vi "Test String To Codepoint Array.vi"(8 "error in (no error)":errorcluster) -> (0 "error out":errorcluster, 3 "Pass?":bool)   [LabVIEW 2020]
uses:
  G-Unicode/Unicode/Controls/String Encoding.ctl
  G-Unicode/Types/UTF-8 String/UTF-8 String.lvclass/UTF-8 String.ctl
  d266910f-e59a-4c09-865c-c189f5680185.vi
  58239b0c-a6dd-4acd-8f33-f6b76af51e62.vi
  18196cac-081f-454a-8ece-801215b674c5.vi
  G-Unicode/Unicode/Encode String.vi
  d266910f-e59a-4c09-865c-c189f5680185.vi/46bf550a-28c6-4dfd-813a-9b0ad34779ef.vi
  G-Unicode/Private/Conversion/String as Encoded String.vi
  G-Unicode/Private/Conversion/Polymorphic VIs/String as Encoded String (UTF-8 String).vi
  G-Unicode/Types/UTF-8 String/Write Encoded UTF-8 String.vi
  G-Unicode/Private/Library/gu_string_to_codepoint_array.vi
  G-Unicode/Private/Library/gu_codepoint_array_to_string.vi
  G-Unicode/Private/Conversion/Polymorphic VIs/String as Encoded String (LabVIEW String).vi
  G-Unicode/Private/Conversion/Text to UTF-8.vi
  G-Unicode/Private/Conversion/Polymorphic VIs/Text to UTF-8 (LabVIEW String).vi
  G-Unicode/Private/Conversion/Encoded UTF-8 String to Encoded UTF-16LE String.vi
  G-Unicode/Unicode/SubVIs/UTF-16 Byte Swap.vi
  G-Unicode/Private/Conversion/UTF-8 to Text.vi
  G-Unicode/Private/Conversion/Polymorphic VIs/UTF-8 to Text (LabVIEW String).vi
  G-Unicode/Private/Conversion/Encoded UTF-16LE String to Encoded UTF-8 String.vi
  G-Unicode/Unicode/Prepend BOM.vi
  G-Unicode/Types/UTF-8 String/Read Encoded UTF-8 String.vi
  G-Unicode/Private/Library/Result To Error.vi
  G-Unicode/Private/Library/gu_string_to_codepoint_array.vi/5c793459-c97f-49eb-b871-f007f412847a.vi
  G-Unicode/Private/Memory/Copy String.vi
  G-Unicode/Unicode/SubVIs/Byte Order Marks.vi
  G-Unicode/Unicode/Detect BOM.vi
  G-Unicode/Private/Library/gu_free.vi
  G-Unicode/Private/Library/gu_string_to_codepoint_array.vi/5c793459-c97f-49eb-b871-f007f412847a.vi/bf7dd0c3-7326-468c-a5c4-9eb034008d84.vi
  G-Unicode/Private/Memory/Copy String.vi/4d47babd-4a2d-4eb7-b91b-7e707d692665.vi
  <vilib>/Utility/error.llb/Error Cluster From Error Code.vi
  G-Unicode/Unicode/Detect String Encoding.vi
  G-Unicode/Types/UTF-8 String/UTF-8 String.lvclass
  G-Unicode/G-Unicode.lvlib
  e3aa35ab-ae09-4e00-bfb9-de3f364217f6.vi
  78ebccf6-81a8-4018-ac4e-97445d2cc37d.vi
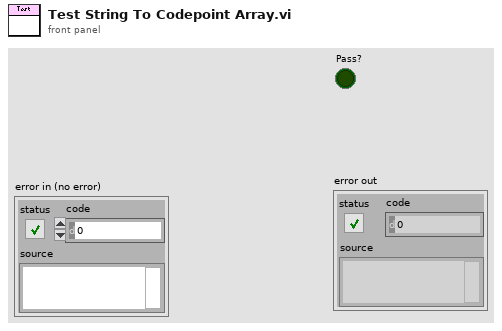
[diagram p1: front panel]
types:
  T1 = typedef "G-Unicode.lvlib/String Encoding.ctl" = enum16{"ANSI", "UTF-8", "UTF-16LE", "UTF-16BE", "Unknown"}
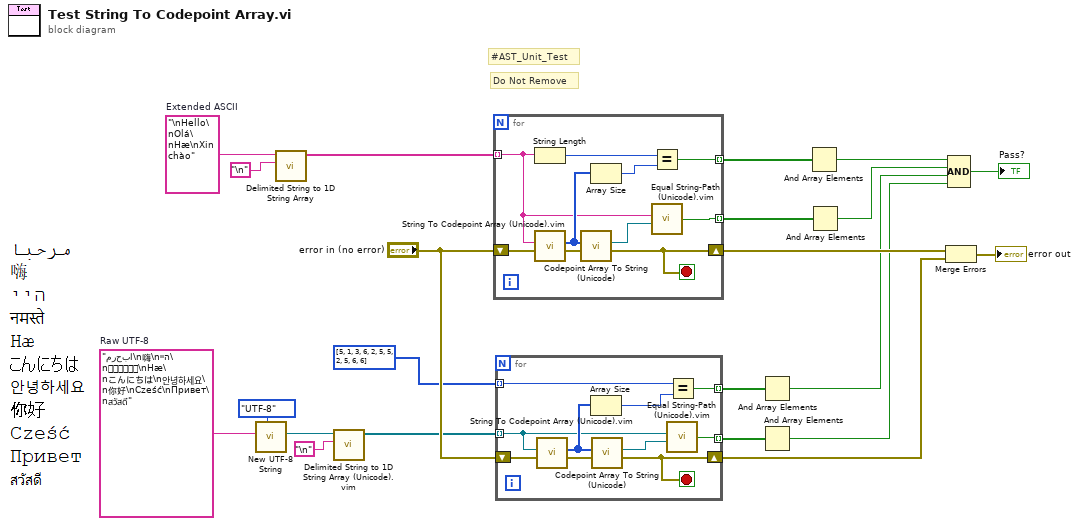
[diagram p0: block diagram]
diagram:
  w12 = "\nHello\nOlá\nHæ\nXin chào"  # Extended ASCII
  w2 = "مرحبا\n嗨\nהיי\nनमस्ते\nHæ\nこんにちは\n안녕하세요\n你好\nCześć\nПривет\nสวัสดี"  # Raw UTF-8
  # "Do Not Remove"
  # "#AST_Unit_Test"
  n1 = call "New UTF-8 String.vi"("Input Encoding (ANSI)"=String_Encoding."UTF-8", "String"=w2) -> ("UTF-8 String"=w4:refnum<class "UTF-8 String.lvclass">)  [unwired: 8 in, 1 out]
  n2 = call <vilib>:"Delimited String to 1D String Array.vi"("delimiter"="\n", "delimited string"=w12) -> ("string array"=w11:string[])  [unwired: 9 in]
  n3 = call "Delimited String to 1D String Array (Unicode).vim"("Delimiter (tab)"="\n", "Delimited String"=w4) -> ("String Array"=w1:refnum<class "UTF-8 String.lvclass">[])  [unwired: 8 in, 1 out]
  n4 = for {
    tunnel: [w32] -> w19 mode=indexing
    shift-right: [w26] -> w22
    shift-left: "error in (no error)" -> [w30]
    tunnel: w11 -> [w24] mode=indexing
    tunnel: [w23] -> w7 mode=indexing
    stop <- w26 stop-if-true
    n5 = String Length(string=w24) -> (length=w31:i32)
    n6 = call "String To Codepoint Array (Unicode).vim"("error in"=w30, "String"=w24) -> ("error out"=w28:errorcluster, "Codepoint Array"=w27:i32[])  [unwired: 8 in]
    n7 = call "Codepoint Array To String (Unicode).vi"("error in"=w28, "Codepoint Array"=w27) -> ("error out"=w26:errorcluster, "String"=w25:refnum<class "UTF-8 String.lvclass">)  [unwired: 8 in]
    n8 = Array Size(array=w27) -> (size(s)=w29:i32)
    n9 = Equal?(x=w31, y=w29) -> (x = y?=w32:bool)
    n10 = call "Equal String-Path (Unicode).vim"("y"=w25, "x"=w24) -> ("Equal?"=w23:bool)  [unwired: 7 in, 1 out]
  }
  n11 = for {
    tunnel: w1 -> [w35] mode=indexing
    tunnel: [w42] -> w17 mode=indexing
    shift-right: [w36] -> w15
    shift-left: "error in (no error)" -> [w40]
    tunnel: i32[] [5, 1, 3, 6, 2, 5, 5, 2, 5, 6, 6] ("Array") -> [w41] mode=indexing
    tunnel: [w33] -> w9 mode=indexing
    stop <- w36 stop-if-true
    n12 = call "String To Codepoint Array (Unicode).vim"("error in"=w40, "String"=w35) -> ("error out"=w37:errorcluster, "Codepoint Array"=w38:i32[])  [unwired: 8 in]
    n13 = Array Size(array=w38) -> (size(s)=w39:i32)
    n14 = call "Codepoint Array To String (Unicode).vi"("error in"=w37, "Codepoint Array"=w38) -> ("error out"=w36:errorcluster, "String"=w34:refnum<class "UTF-8 String.lvclass">)  [unwired: 8 in]
    n15 = call "Equal String-Path (Unicode).vim"("y"=w34, "x"=w35) -> ("Equal?"=w33:bool)  [unwired: 7 in, 1 out]
    n16 = Equal?(x=w41, y=w39) -> (x = y?=w42:bool)
  }
  n17 = And Array Elements(Boolean array=w17) -> (logical AND=w16:bool)
  n18 = And Array Elements(Boolean array=w9) -> (logical AND=w8:bool)
  n19 = And Array Elements(Boolean array=w19) -> (logical AND=w18:bool)
  n20 = And Array Elements(Boolean array=w7) -> (logical AND=w6:bool)
  n21 = Merge Errors(w22, w15) -> (→"error out":errorcluster)
  n22 = Compound Arithmetic op=AND(w18, w6, w16, w8) -> (→"Pass?":bool)
